vi "check_if_file_exists.vi"(8 "error_in":errorcluster, 11 "file_path_in":path) -> (0 "error_out":errorcluster, 3 "file_path_out":path)   [LabVIEW 2020]
uses:
  AULocalize/SubVIs/Get Localized Phrase Compact Interface 0D.vi
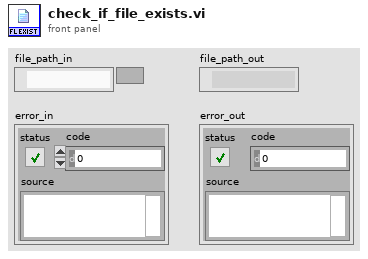
[diagram p1: front panel]
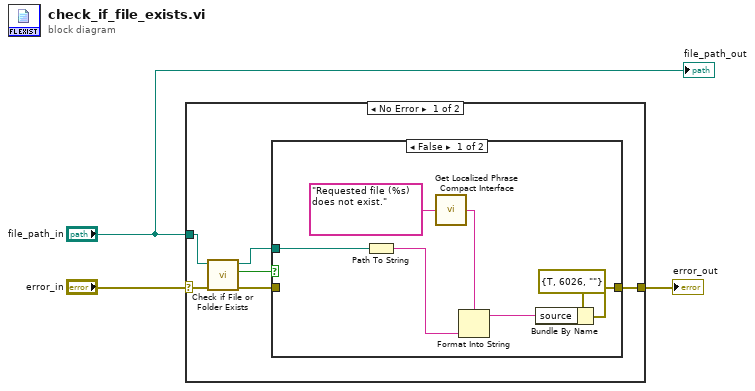
[diagram p0: block diagram]
diagram:
  n1 = case shown="No Error" "error_in" {
    selector: "error_in" -> [w4 w18]
    tunnel: [w6 w18] -> w3
    tunnel: "file_path_in" -> [w5 _]
    frame No Error {
      n2 = call <vilib>:"Check if File or Folder Exists.vi"("error in (no error)"=w4, "path"=w5) -> ("error out"=w9:errorcluster, "file or folder exists?"=w7:bool, "dup path"=w8:path)  [unwired: 7 in]
      n3 = case shown="False" w7 {
        tunnel: [w16 w17] -> w6
        tunnel: w8 -> [w15 _]
        tunnel: w9 -> [_ w17]
        frame False {
          n4 = Path To String(path=w15) -> (string=w13:string)
          n5 = call-poly "Get Localized Phrase Compact Interface.vi"("Key"="Requested file (%s) does not exist." ("format string")) -> ("Translated Phrase"=w10:string)
          n6 = Format Into String(format string=w10, w13) -> (resulting string=w12:string)  [unwired: 2 in, 1 out]
          n7 = Bundle By Name(cluster=errorcluster {"status"=TRUE, "code"=6026, "source"=""} ("error out"), "source"=w12) -> (w16:errorcluster)
        }
        frame True {
        }
      }
    }
    frame Error {
    }
  }
  "error_out" <- w3
  "file_path_out" <- "file_path_in"
